vi "Charger_Close.vi"(4 "error in":errorcluster, 7 "address":refnum<visa-resource-name>="COM7") -> (0 "error out":errorcluster)   [LabVIEW 2020]
doc: "This function closes the Charger Test Set serial port"
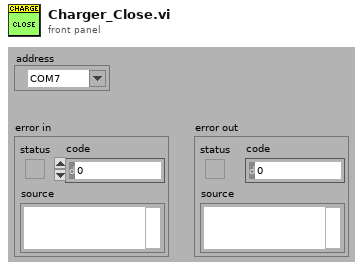
[diagram p1: front panel]
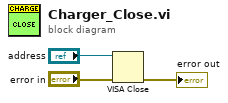
[diagram p0: block diagram]
diagram:
  n1 = VISA Close(VISA resource name="address", error in (no error)="error in") -> (error out=→"error out":errorcluster)
